vi "PH_Trendviewer_Powermeter.Data Collector.vi"(0 "i ref in":refnum<vi>, 2 "Energy [J]":dbl, 5 "error in (no error)":errorcluster) -> (14 "i ref out":refnum<vi>, 19 "error out":errorcluster)   [LabVIEW 2014, in "PH_Trendviewer_Powermeter.lvlib"]
doc: "This VI reads the data of the connected image operator."
uses:
  PH_Trendviewer_Powermeter.lvlib
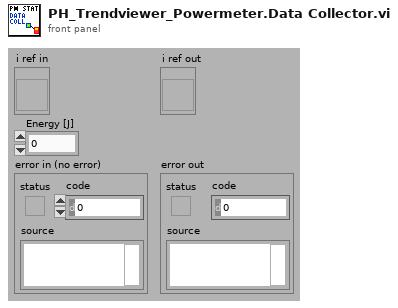
[diagram p1: front panel]
types:
  T1 = typedef "PH_Trendviewer_Powermeter.lvlib/PH_Trendviewer_Powermeter.i attribute.ctl" = cluster{"GUI Refs ":cluster{"Status":refnum<vi>, "Result Graph":refnum<vi>, "Mean Data":refnum<vi>, "Std Dev Data":refnum<vi>, "Dummy Mean":refnum<vi>, "Dummy Std Dev":refnum<vi>, "Export Data":refnum<vi>, "Stat or Trend":refnum<vi>, "Delete":refnum<vi>, "Powermeter":refnum<vi>, "Start":refnum<vi>}, "Powermeter":string, "Stat or Trend":bool, "Start":bool, "Data":cluster{"Time Stamp":timestamp, "Energy [J]":dbl}[], "Datasets strored":i32, "Dataarray Size":i32}
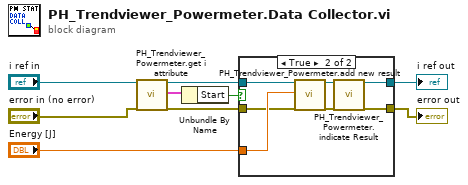
[diagram p0: block diagram]
diagram:
  n1 = call "PH_Trendviewer_Powermeter.get i attribute.vi"("i ref in"="i ref in", "error in (no error)"="error in (no error)") -> ("i ref out"=w3:refnum<vi>, "i attribute"=w2:T1, "error out"=w5:errorcluster)  [unwired: 15 in]
  n2 = Unbundle By Name(w2) -> ("Start"=w1:bool)
  n3 = case shown="True" w1 {
    tunnel: [w11 w18] -> w9
    tunnel: [w10 w17] -> w8
    tunnel: "Energy [J]" -> [_ w16]
    tunnel: w5 -> [w10 w13]
    tunnel: w3 -> [w11 w12]
    frame False {
    }
    frame True {
      n4 = call "PH_Trendviewer_Powermeter.add new result.vi"("i ref in"=w12, "Energy [J]"=w16, "error in (no error)"=w13) -> ("i ref out"=w14:refnum<vi>, "error out"=w15:errorcluster)  [unwired: 15 in]
      n5 = call "PH_Trendviewer_Powermeter.indicate Result.vi"("i ref in"=w14, "error in (no error)"=w15) -> ("i ref out"=w18:refnum<vi>, "error out"=w17:errorcluster)  [unwired: 16 in]
    }
  }
  "i ref out" <- w9
  "error out" <- w8
